vi "Command_fire_cmd.vi"(6 "error in":errorcluster, 9 "command line":string="python C:\\\\Users\\\\vvdn\\\\Downloads\\\\frame_cap.py") -> (0 "error out":errorcluster, 2 "standard error":string, 3 "standard output":string)   [LabVIEW 2019]
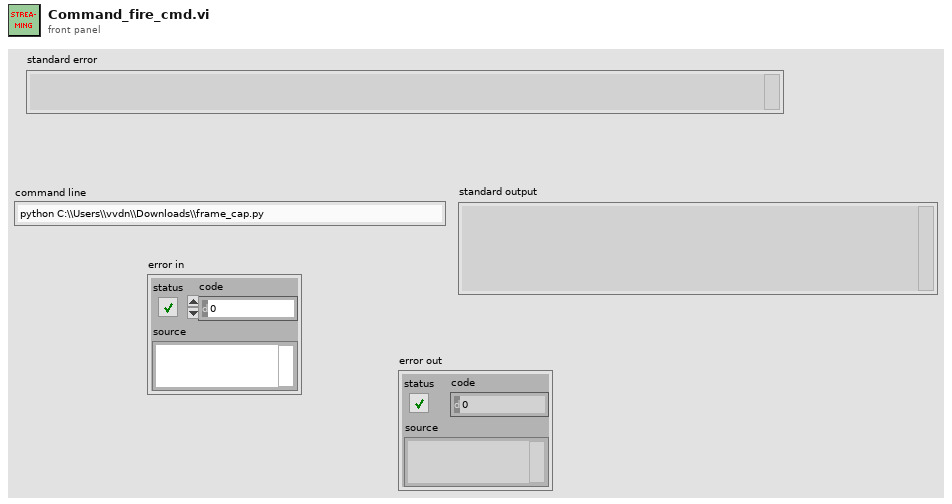
[diagram p1: front panel]
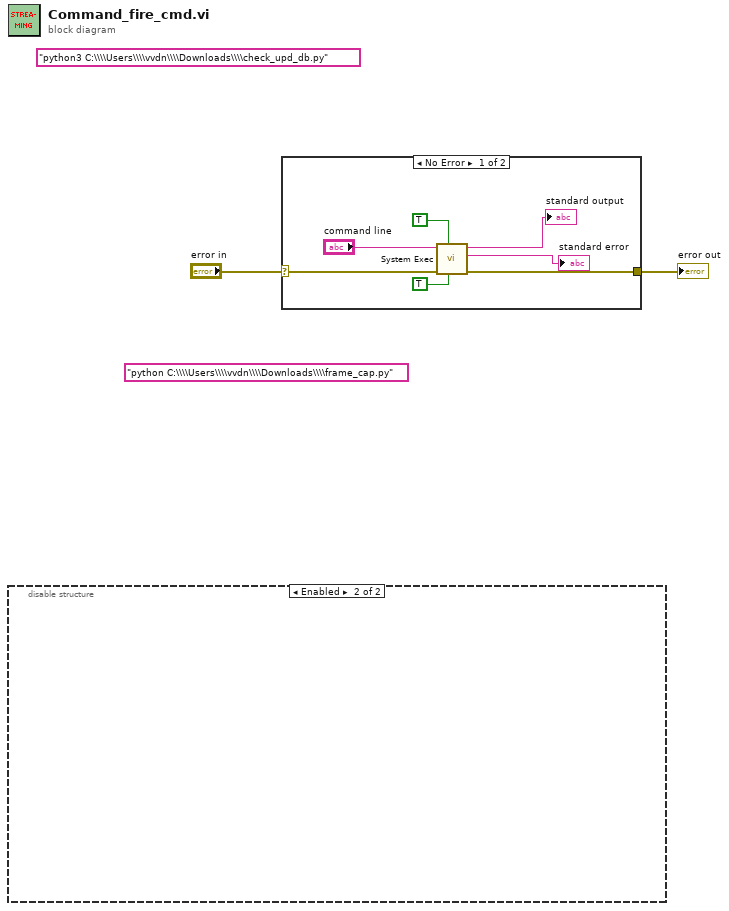
[diagram p0: block diagram]
diagram:
  (unwired) "python3 C:\\\\Users\\\\vvdn\\\\Downloads\\\\check_upd_db.py"
  (unwired) "python C:\\\\Users\\\\vvdn\\\\Downloads\\\\frame_cap.py" ("command line")
  n1 = disable-structure shown="Enabled" {
    frame Disabled {
    }
    frame Enabled {
    }
  }
  n2 = case shown="No Error" "error in" {
    selector: "error in" -> [w5 w10]
    tunnel: [w6 w10] -> w2
    frame No Error {
      n3 = call <vilib>:"System Exec.vi"("run minimized? (F)"=TRUE, "wait until completion? (T)"=TRUE, "error in (no error)"=w5, "command line"="command line") -> ("error out"=w6:errorcluster, "standard error"=→"standard error":string, "standard output"=→"standard output":string)  [unwired: 4 in, 1 out]
    }
    frame Error {
    }
  }
  "error out" <- w2
